vi "SW_Convert_data_from_old_format_save_2.vi"(7 "Time Stamp in":timestamp format="%<%.0X\n%x>T", 8 "error in (no error)":errorcluster, 9 "File name":string="Loaded file of previous version", 10 "Researcher name":string="Researcher", 11 "Loaded data in":T2) -> (0 "error out":errorcluster, 3 "Loaded data out":T1)   [LabVIEW 2018, in "Tracker.lvlib"]
uses:
  Tracker.lvlib
  Controls/CTL_Loaded_data_output_(offline).ctl
  Controls/CTL_Settings_cluster.ctl
  Controls/CTL_Histogram_parameters.ctl
  Controls/CTL_Filter_selector.ctl
  Controls/CTL_Acquisition_speed_selector.ctl
  Controls/CTL_Segmented_plot_parameters_2.ctl
  Libraries/Cage Diagram/Typedefs/CTL_Cage_type.ctl
  Controls/CTL_Cage_all_segmentation_params_set.ctl
  Controls/CTL_IO_params_cluster.ctl
  Controls/CTL_Conditions_Array.ctl
  Controls/CTL_Conditions_Cluster.ctl
  Controls/CTL_Condition_type.ctl
  Controls/CTL_Comparison_type.ctl
  Controls/CTL_Validity_check_criteria.ctl
  Controls/CTL_Response_info.ctl
  Controls/CTL_Condition_response_type.ctl
  Controls/CTL_Reponse_port_info.ctl
  Controls/CTL_Calibration_parameters.ctl
  Controls/CTL_Dispenser_calibration_info.ctl
  Controls/CTL_Segmented_plot_parameters_2_(round_d1).ctl
  <vilib>/Analysis/baseanly.llb/Mean (DBL).vi
  Common_Resources.lvlib
  <vilib>/Analysis/NI_AALBase.lvlib
  Libraries/Cage Diagram/Cage Diagram.lvlib
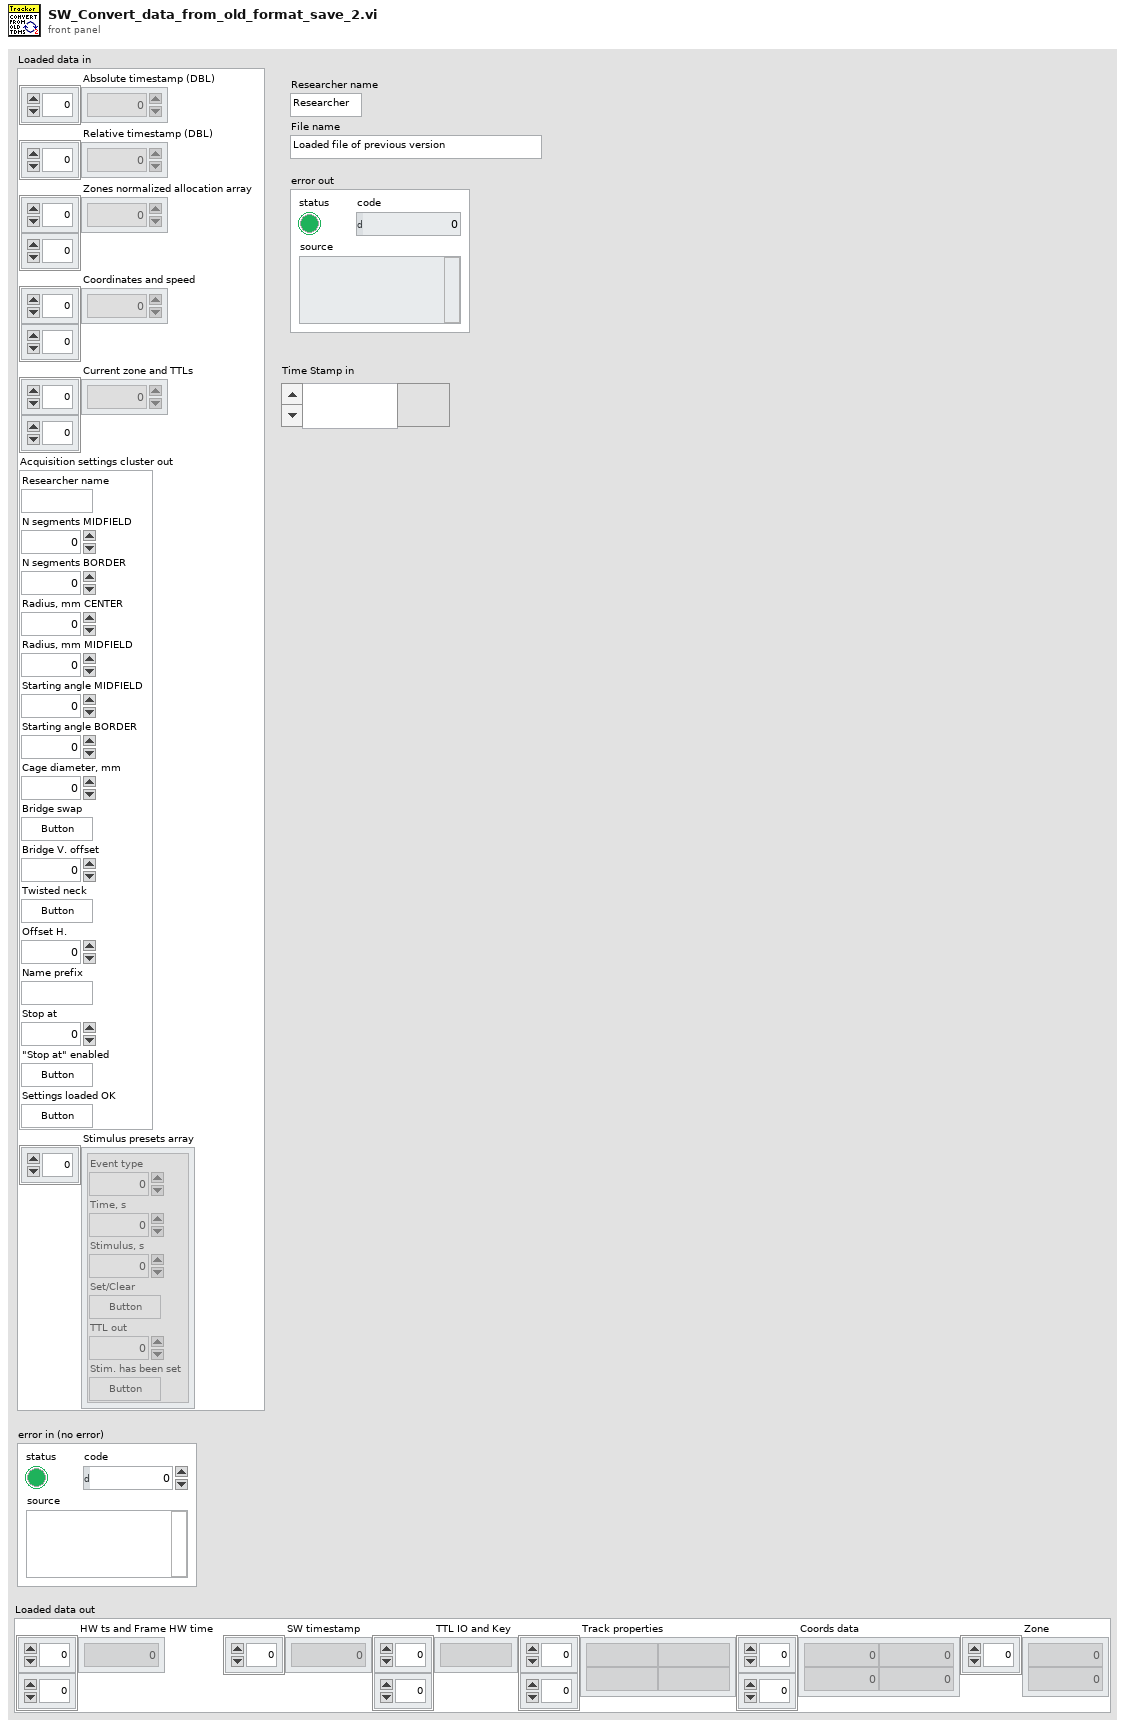
[diagram p1: front panel]
types:
  T1 = typedef "Common_Resources.lvlib/CTL_Loaded_data_output_(offline).ctl" = cluster{"HW ts and Frame HW time":u32[][], "SW timestamp":dbl[], "TTL IO and Key":string[][], "Track properties":string[][], "Coords data":dbl[][], "Zone":i8[]}
  T2 = cluster{"Absolute timestamp (DBL)":dbl[], "Relative timestamp (DBL)":dbl[], "Zones normalized allocation array":dbl[][], "Coordinates and speed":dbl[][], "Current zone and TTLs":u8[][], "Acquisition settings cluster out":cluster{"Researcher name":string, "N segments MIDFIELD":u8, "N segments BORDER":u8, "Radius, mm CENTER":u16, "Radius, mm MIDFIELD":u16, "Starting angle MIDFIELD":i16, "Starting angle BORDER":i16, "Cage diameter, mm":u16, "Bridge swap":bool, "Bridge V. offset":sgl, "Twisted neck":bool, "Offset H.":sgl, "Name prefix":string, "Stop at":dbl, "\"Stop at\" enabled":bool, "Settings loaded OK":bool}, "Stimulus presets array":cluster{"Event type":u16, "Time, s":sgl, "Stimulus, s":sgl, "Set/Clear":bool, "TTL out":u16, "Stim. has been set":bool}[]}
  T3 = typedef "Common_Resources.lvlib/CTL_Segmented_plot_parameters_2_(round_d1).ctl" = cluster{"Cage diameter, mm":u16, "Starting angle BORDER":i16, "Starting angle MIDFIELD":i16, "Radius, mm MIDFIELD":u16, "Radius, mm CENTER":u16, "N segments BORDER":u8, "N segments MIDFIELD":u8, "R-gap, mm":sgl}
  T4 = typedef "Common_Resources.lvlib/CTL_Segmented_plot_parameters_2.ctl" = cluster{"Sensor board size":enum16{"", "Large"}, "Bridge swap":bool, "Twisted neck":bool, "Bridge H. offset":sgl, "Bridge V. offset":sgl, "Magnets orientation":sgl, "Cage type":T5, "Cage parameters":T6}
  T5 = typedef "Cage Diagram.lvlib/CTL_Cage_type.ctl" = u16
  T6 = typedef "Common_Resources.lvlib/CTL_Cage_all_segmentation_params_set.ctl" = cluster{"Round":variant, "Square":variant, "Donut-maze":variant, "T-maze":variant, "Sociability-maze":variant}
  T7 = typedef "Common_Resources.lvlib/CTL_Settings_cluster.ctl" = cluster{"Defaults":cluster{"Default User":dbl, "VISA Resource Name ":string, "Histogram parameters":T8}, "Recording and saving":cluster{"Researcher name":string, "Name prefix":string, "Data post-processing":T9, "Stop at":dbl, "\"Stop at\" enabled":bool, "Default save folder path":path, "Acquisition FPS":T10}, "Geometry":T4, "IO parameters":T11, "Conditions presets array":T12, "Calibration parameters":T20, "Settings loaded OK":bool}
  T8 = typedef "Common_Resources.lvlib/CTL_Histogram_parameters.ctl" = cluster{"max":dbl, "min":dbl, "# bins":i32, "threshold":dbl, "thr. type":enum16{"higher accepted", "lower accepted"}}
  T9 = typedef "Common_Resources.lvlib/CTL_Filter_selector.ctl" = cluster{"Filter type":enum16{"None", "Savitzky-Golay"}, "Length":i32, "Order":i32}
  T10 = typedef "Common_Resources.lvlib/CTL_Acquisition_speed_selector.ctl" = enum16{"Max", "Optimal", "Eco"}
  T11 = typedef "Common_Resources.lvlib/CTL_IO_params_cluster.ctl" = cluster{"IO general config.":u16, "IO 1 configuration":u16, "IO 2 configuration":u16, "IO 3 configuration":u16, "IO 4 configuration":u16, "Activate ext. RS-232":u16, "IO inversion config.":u16, "Sync capability":u8}
  T12 = typedef "Common_Resources.lvlib/CTL_Conditions_Array.ctl" = T13[]
  T13 = typedef "Common_Resources.lvlib/CTL_Conditions_Cluster.ctl" = cluster{"Enabled":bool, "Name":string, "Specifier(s)":cluster{"Specifier enabled":bool, "Condition type":T14, "Comparison type":T15, "Value":dbl, "Validity criteria(s)":cluster{"V. check enabled":bool, "Criteria":T16, "Validity value":dbl}[]}[], "Response":T17, "Has been set":bool}
  T14 = typedef "Common_Resources.lvlib/CTL_Condition_type.ctl" = enum16{"Speed", "Zone", "Angle to wall"}
  T15 = typedef "Common_Resources.lvlib/CTL_Comparison_type.ctl" = enum16{"Less", "Less or Equal", "Equal", "Greater or Equal", "Greater", "Not Equal"}
  T16 = typedef "Common_Resources.lvlib/CTL_Validity_check_criteria.ctl" = enum16{"Running bout (seconds)", "Running bout (meters)"}
  T17 = typedef "Common_Resources.lvlib/CTL_Response_info.ctl" = cluster{"Response type":T18, "TTL port":T19, "TTL pulse length, ms":dbl}
  T18 = typedef "Common_Resources.lvlib/CTL_Condition_response_type.ctl" = enum16{"None", "Air puff", "Liquid reward", "TTL pulse", "TTL pulse (ubr)", "TTL signal"}
  T19 = typedef "Common_Resources.lvlib/CTL_Reponse_port_info.ctl" = enum16{"Port 1", "Port 2", "Port 3", "Port 4"}
  T20 = typedef "Common_Resources.lvlib/CTL_Calibration_parameters.ctl" = cluster{"Timing calibration sw/hw":dbl, "True FPS":dbl, "True frame time, s":dbl, "Disp. calibration info":T21}
  T21 = typedef "Common_Resources.lvlib/CTL_Dispenser_calibration_info.ctl" = cluster{"Channel":u8, "Speed, µl per ms":dbl}[]
  T22 = cluster{"Researcher name":string, "N segments MIDFIELD":u8, "N segments BORDER":u8, "Radius, mm CENTER":u16, "Radius, mm MIDFIELD":u16, "Starting angle MIDFIELD":i16, "Starting angle BORDER":i16, "Cage diameter, mm":u16, "Bridge swap":bool, "Bridge V. offset":sgl, "Twisted neck":bool, "Offset H.":sgl, "Name prefix":string, "Stop at":dbl, "\"Stop at\" enabled":bool, "Settings loaded OK":bool}
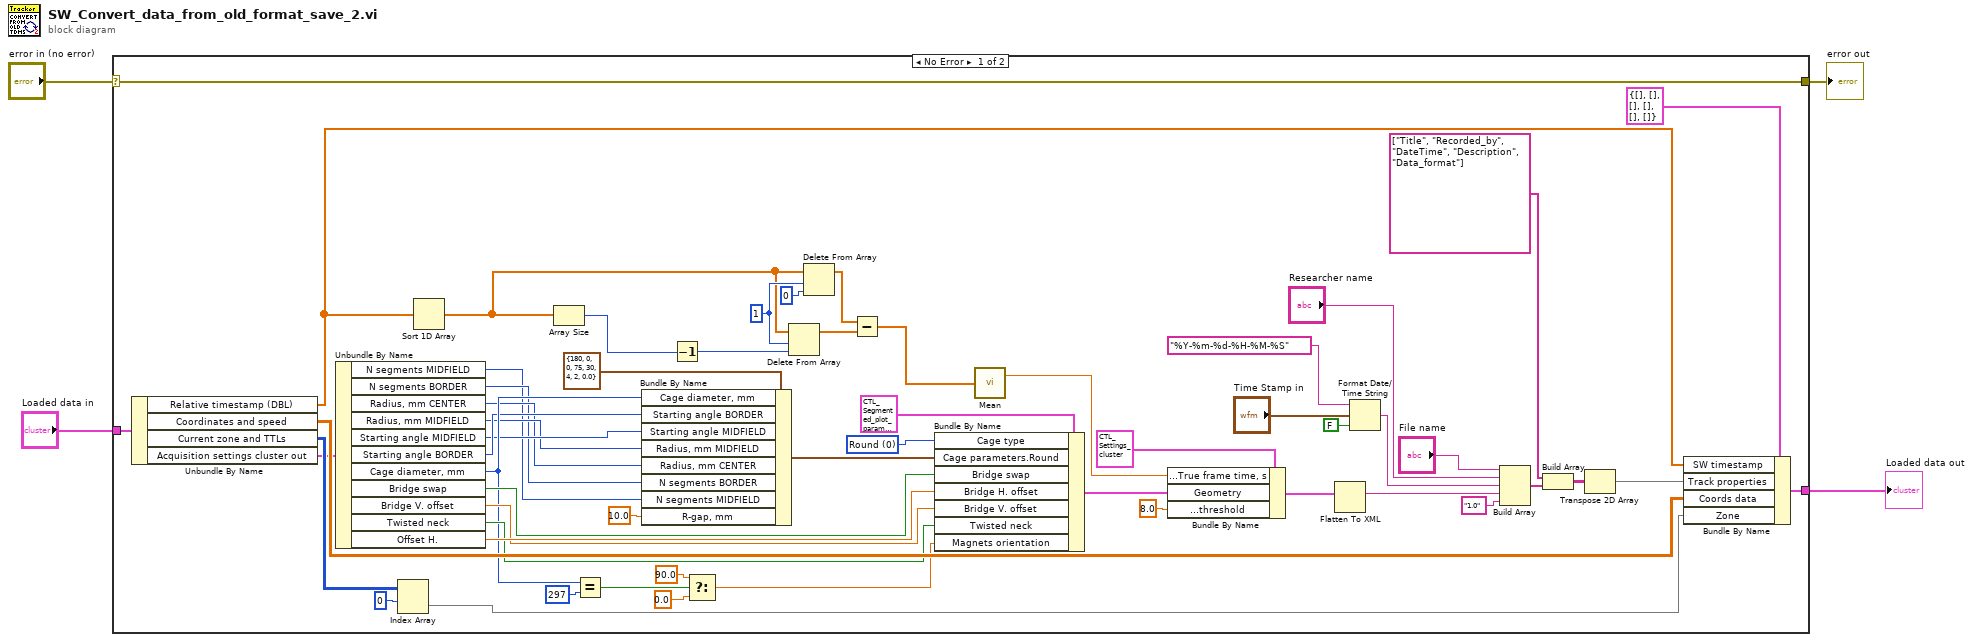
[diagram p0: block diagram]
diagram:
  n1 = case shown="No Error" "error in (no error)" {
    selector: "error in (no error)" -> [w5 w61]
    tunnel: "Loaded data in" -> [w60 _]
    tunnel: [w46 _] -> w3
    tunnel: [w5 w61] -> w1
    frame No Error {
      w17 = T5 0 items=["Round", "Square", "Donut-maze", "T-maze", "Sociability maze", ""] ("Cage type")
      w43 = 1 ("length")
      n2 = Unbundle By Name(w60) -> ("Relative timestamp (DBL)"=w38:dbl[], "Coordinates and speed"=w57:dbl[][], "Current zone and TTLs"=w56:u8[][], "Acquisition settings cluster out"=w52:T22)
      n3 = Unbundle By Name(w52) -> ("N segments MIDFIELD"=w7:u8, "N segments BORDER"=w8:u8, "Radius, mm CENTER"=w9:u16, "Radius, mm MIDFIELD"=w10:u16, "Starting angle MIDFIELD"=w11:i16, "Starting angle BORDER"=w12:i16, "Cage diameter, mm"=w14:u16, "Bridge swap"=w51:bool, "Bridge V. offset"=w48:sgl, "Twisted neck"=w49:bool, "Offset H."=w50:sgl)
      n4 = Index Array(array=w56, index (row)=0) -> (element=w54:u8[])  [unwired: 1 in]
      n5 = Sort 1D Array(array=w38) -> (sorted array=w37:dbl[])
      n6 = Array Size(array=w37) -> (size(s)=w44:i32)
      n7 = Equal?(x=w14, y=u16 297) -> (x = y?=w21:bool)
      n8 = Bundle By Name(cluster=T3 {"Cage diameter, mm"=180, "Starting angle BORDER"=0, "Starting angle MIDFIELD"=0, "Radius, mm MIDFIELD"=75, "Radius, mm CENTER"=30, "N segments BORDER"=4, "N segments MIDFIELD"=2, "R-gap, mm"=0.0} ("Radial segmentation parameters"), "Cage diameter, mm"=w14, "Starting angle BORDER"=w12, "Starting angle MIDFIELD"=w11, "Radius, mm MIDFIELD"=w10, "Radius, mm CENTER"=w9, "N segments BORDER"=w8, "N segments MIDFIELD"=w7, "R-gap, mm"=sgl 10.0) -> (w15:T3)
      n9 = Decrement(x=w44) -> (x-1=w42:i32)
      n10 = Select(t=90.0, s=w21, f=0.0) -> (s? t:f=w20:dbl)
      n11 = Delete From Array(array=w37, length=w43, index=w42) -> (array with subset deleted=w40:dbl[])  [unwired: 1 out]
      n12 = Delete From Array(array=w37, length=w43, index=0) -> (array with subset deleted=w41:dbl[])  [unwired: 1 out]
      n13 = Subtract(x=w41, y=w40) -> (x-y=w39:dbl[])
      n14 = Bundle By Name(cluster=T4 {"Sensor board size"=enum."", "Bridge swap"=FALSE, "Twisted neck"=FALSE, "Bridge H. offset"=0.0, "Bridge V. offset"=0.0, "Magnets orientation"=0.0, "Cage type"=0, "Cage parameters"={"Round"=variant, "Square"=variant, "Donut-maze"=variant, "T-maze"=variant, "Sociability-maze"=variant}} ("Geometry"), "Cage type"=w17, "Cage parameters.Round"=w15, "Bridge swap"=w51, "Bridge H. offset"=w50, "Bridge V. offset"=w48, "Twisted neck"=w49, "Magnets orientation"=w20) -> (w6:T4)
      n15 = call-poly <vilib>:"Mean.vi"("X"=w39) -> ("mean"=w36:dbl)  [unwired: 1 out]
      n16 = Bundle By Name(cluster=T7 {"Defaults"={"Default User"=0.0, "VISA Resource Name "="Tracker", "Histogram parameters"={"max"=300.0, "min"=0.0, "# bins"=10, "threshold"=8.0, "thr. type"=enum."higher accepted"}}, "Recording and saving"={"Researcher name"="Researcher", "Name prefix"="Track", "Data post-processing"={"Filter type"=enum."Savitzky-Golay", "Length"=31, "Order"=3}, "Stop at"=0.0, "\"Stop at\" enabled"=FALSE, "Default save folder path"=path "", "Acquisition FPS"=enum."Max"}, "Geometry"={"Sensor board size"=enum."", "Bridge swap"=FALSE, "Twisted neck"=FALSE, "Bridge H. offset"=0.0, "Bridge V. offset"=0.0, "Magnets orientation"=180.0, "Cage type"=0, "Cage parameters"={"Round"=variant(i16 0), "Square"=variant(u16 30), "Donut-maze"=variant(u16 75), "T-maze"=variant(u8 2), "Sociability-maze"=variant(u8 4)}}, "IO parameters"={"IO general config."=12, "IO 1 configuration"=1, "IO 2 configuration"=1, "IO 3 configuration"=0, "IO 4 configuration"=0, "Activate ext. RS-232"=0, "IO inversion config."=0, "Sync capability"=1}, "Conditions presets array"=[{"Enabled"=FALSE, "Name"="", "Specifier(s)"=[], "Response"={"Response type"=enum."Air puff", "TTL port"=enum."Port 1", "TTL pulse length, ms"=0.0}, "Has been set"=FALSE}, {"Enabled"=FALSE, "Name"="", "Specifier(s)"=[], "Response"={"Response type"=enum."Air puff", "TTL port"=enum."Port 1", "TTL pulse length, ms"=0.0}, "Has been set"=FALSE}, {"Enabled"=FALSE, "Name"="", "Specifier(s)"=[], "Response"={"Response type"=enum."Air puff", "TTL port"=enum."Port 1", "TTL pulse length, ms"=0.0}, "Has been set"=FALSE}, {"Enabled"=FALSE, "Name"="", "Specifier(s)"=[], "Response"={"Response type"=enum."Air puff", "TTL port"=enum."Port 1", "TTL pulse length, ms"=0.0}, "Has been set"=FALSE}, {"Enabled"=FALSE, "Name"="", "Specifier(s)"=[], "Response"={"Response type"=enum."Air puff", "TTL port"=enum."Port 1", "TTL pulse length, ms"=0.0}, "Has been set"=FALSE}, {"Enabled"=FALSE, "Name"="", "Specifier(s)"=[], "Response"={"Response type"=enum."Air puff", "TTL port"=enum."Port 1", "TTL pulse length, ms"=0.0}, "Has been set"=FALSE}, {"Enabled"=FALSE, "Name"="", "Specifier(s)"=[], "Response"={"Response type"=enum."Air puff", "TTL port"=enum."Port 1", "TTL pulse length, ms"=0.0}, "Has been set"=FALSE}, {"Enabled"=FALSE, "Name"="", "Specifier(s)"=[], "Response"={"Response type"=enum."Air puff", "TTL port"=enum."Port 1", "TTL pulse length, ms"=0.0}, "Has been set"=FALSE}, {"Enabled"=FALSE, "Name"="", "Specifier(s)"=[], "Response"={"Response type"=enum."Air puff", "TTL port"=enum."Port 1", "TTL pulse length, ms"=0.0}, "Has been set"=FALSE}, {"Enabled"=FALSE, "Name"="", "Specifier(s)"=[], "Response"={"Response type"=enum."Air puff", "TTL port"=enum."Port 1", "TTL pulse length, ms"=0.0}, "Has been set"=FALSE}, {"Enabled"=FALSE, "Name"="", "Specifier(s)"=[], "Response"={"Response type"=enum."Air puff", "TTL port"=enum."Port 1", "TTL pulse length, ms"=0.0}, "Has been set"=FALSE}, {"Enabled"=FALSE, "Name"="", "Specifier(s)"=[], "Response"={"Response type"=enum."Air puff", "TTL port"=enum."Port 1", "TTL pulse length, ms"=0.0}, "Has been set"=FALSE}, {"Enabled"=FALSE, "Name"="", "Specifier(s)"=[], "Response"={"Response type"=enum."Air puff", "TTL port"=enum."Port 1", "TTL pulse length, ms"=0.0}, "Has been set"=FALSE}, {"Enabled"=FALSE, "Name"="", "Specifier(s)"=[], "Response"={"Response type"=enum."Air puff", "TTL port"=enum."Port 1", "TTL pulse length, ms"=0.0}, "Has been set"=FALSE}], "Calibration parameters"={"Timing calibration sw/hw"=1.0, "True FPS"=80.0, "True frame time, s"=0.0125, "Disp. calibration info"=[]}, "Settings loaded OK"=FALSE} ("Settings cluster"), "Calibration parameters.True frame time, s"=w36, "Geometry"=w6, "Defaults.Histogram parameters.threshold"=8.0) -> (w35:T7)
      n17 = Flatten To XML(anything=w35) -> (xml string=w32:string)
      n18 = Format Date/Time String(time format string (%c)="%Y-%m-%d-%H-%M-%S", seconds (now)="Time Stamp in", UTC format=FALSE) -> (date/time string=w27:string)
      n19 = Build Array("File name", "Researcher name", w27, w32, "1.0" ("element")) -> (w26:string[])
      n20 = Build Array(string[] ["Title", "Recorded_by", "DateTime", "Description", "Data_format"] ("property names"), w26) -> (w25:string[][])
      n21 = Transpose 2D Array(2D array=w25) -> (transposed array=w23:string[][])
      n22 = Bundle By Name(cluster=T1 {"HW ts and Frame HW time"=[], "SW timestamp"=[], "TTL IO and Key"=[], "Track properties"=[], "Coords data"=[], "Zone"=[]} ("Loaded data output"), "SW timestamp"=w38, "Track properties"=w23, "Coords data"=w57, "Zone"=w54) -> (w46:T1)
    }
    frame Error {
    }
  }
  "Loaded data out" <- w3
  "error out" <- w1
